vi "GlobalFlipFlag.vi"() -> ()   [LabVIEW 2010]
panel:
  out "Flip Flag":bool
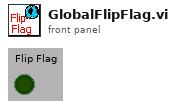
[diagram p1: front panel]
diagram:
